vi "Shutdown Master.vi"(8 "error in":errorcluster, 11 "Serial Master in":refnum<class "Serial Master.lvclass">) -> (0 "error out":errorcluster, 3 "Serial Master out":refnum<class "Serial Master.lvclass">)   [LabVIEW 2012, in "Serial Master.lvclass"]
doc: "This provides an interface for the master to close a connection to the slave."
uses:
  Serial Master.lvclass
  Serial Master.lvclass/Serial Master.ctl
  Read VISA resource name.vi
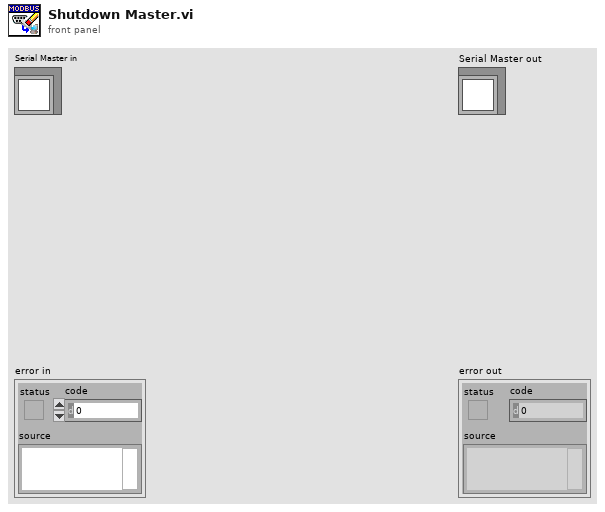
[diagram p1: front panel]
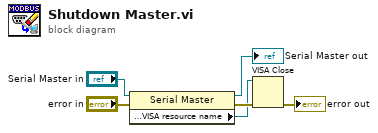
[diagram p0: block diagram]
diagram:
  n1 = property class="Serial Master"(reference="Serial Master in", error in="error in") -> (reference out=→"Serial Master out":refnum<class "Serial Master.lvclass">, error out=w5:errorcluster, "Data Access:VISA resource name"=w4:refnum<visa-resource-name>)
  n2 = VISA Close(VISA resource name=w4, error in (no error)=w5) -> (error out=→"error out":errorcluster)
